vi "Generate GUID.vi"() -> (1 "ToString":string)   [LabVIEW 2020, in "MeasurementTemplate_server.lvlib"]
uses:
  MeasurementTemplate_server.lvlib
panel:
  out "error out":errorcluster
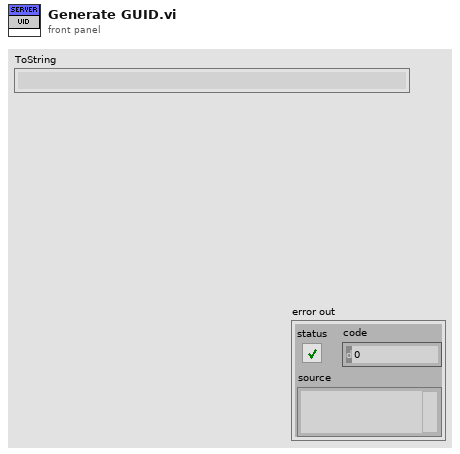
[diagram p1: front panel]
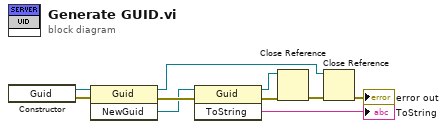
[diagram p0: block diagram]
diagram:
  n1 = constructor class="Guid"() -> (reference out=w4:refnum<k24>, error out=w3:errorcluster)  [unwired: 3 in, 1 out]
  n2 = invoke class="Guid" method="NewGuid"(reference=w4, error in=w3) -> (reference out=w10:refnum<k24>, error out=w7:errorcluster, "NewGuid"=w5:refnum<k24>)  [unwired: 1 in]
  n3 = invoke class="Guid" method="ToString"(reference=w5, error in=w7) -> (reference out=w8:refnum<k24>, error out=w6:errorcluster, "ToString"=→"ToString":string)  [unwired: 1 in]
  n4 = Close Reference(reference=w8, error in (no error)=w6) -> (error out=w9:errorcluster)
  n5 = Close Reference(reference=w10, error in (no error)=w9) -> (error out=→"error out":errorcluster)
